vi "Run_VI.vi"(0 "Application_Directory":path, 11 "Error_In":errorcluster) -> (15 "Error_Out":errorcluster)   [LabVIEW 2021]
doc: "Used to run a vi."
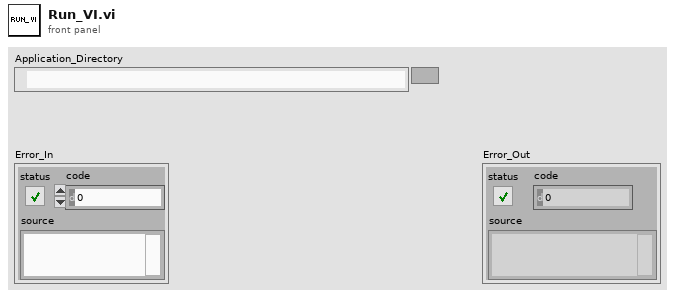
[diagram p1: front panel]
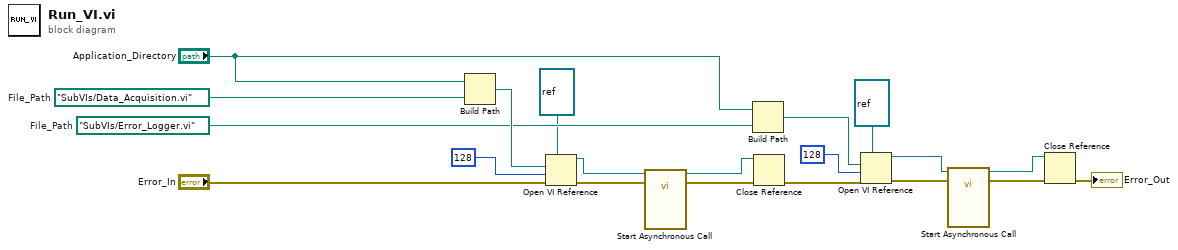
[diagram p0: block diagram]
diagram:
  w15 = path "SubVIs/Error_Logger.vi"  # File_Path
  w18 = path "SubVIs/Data_Acquisition.vi"  # File_Path
  n1 = Build Path(base path="Application_Directory", name or relative path=w18) -> (appended path=w19:path)
  n2 = Open VI Reference(type specifier VI Refnum (for type only)=refnum<vi> refnum, vi path=w19, options=128, error in (no error)="Error_In") -> (vi reference=w10:refnum<vi>, error out=w12:errorcluster)  [unwired: 2 in]
  n3 = call-by-ref "Start Asynchronous Call"(reference=w10, error in=w12) -> (reference out=w9:refnum<vi>, error out=w11:errorcluster)  [unwired: 15 in, 1 out]
  n4 = Build Path(base path="Application_Directory", name or relative path=w15) -> (appended path=w16:path)
  n5 = Close Reference(reference=w9, error in (no error)=w11) -> (error out=w17:errorcluster)
  n6 = Open VI Reference(type specifier VI Refnum (for type only)=refnum<vi> refnum, vi path=w16, options=128, error in (no error)=w17) -> (vi reference=w5:refnum<vi>, error out=w7:errorcluster)  [unwired: 2 in]
  n7 = call-by-ref "Start Asynchronous Call"(reference=w5, error in=w7) -> (reference out=w3:refnum<vi>, error out=w6:errorcluster)  [unwired: 14 in, 2 out]
  n8 = Close Reference(reference=w3, error in (no error)=w6) -> (error out=→"Error_Out":errorcluster)
